vi "Write Current State.vi"(10 "Current State":refnum<class "state.lvclass">, 11 "statemachine in":refnum<class "statemachine.lvclass">) -> (3 "statemachine out":refnum<class "statemachine.lvclass">)   [LabVIEW 2020, in "eos.lvlib" / "statemachine.lvclass"]
uses:
  statemachine.lvclass
  interfaces/state/state.lvclass
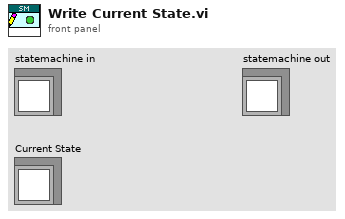
[diagram p1: front panel]
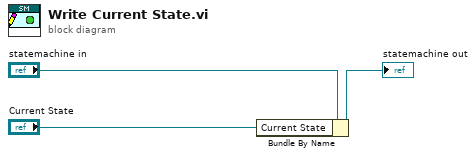
[diagram p0: block diagram]
diagram:
  n1 = Bundle By Name(cluster="statemachine in", "Current State"="Current State") -> (→"statemachine out":refnum<class "statemachine.lvclass">)
